vi "REx - Send Command.vi"(0 "Remote Connection Handle in":T2, 7 "Command Data Element in":T1, 11 "error in (no error)":errorcluster) -> (4 "Remote Connection Handle out":T2, 8 "Command Data Element out":T1, 15 "error out":errorcluster)   [LabVIEW 2012, in "REx.lvlib" / "REx - CMD_TEMPLATE.lvclass"]
uses:
  REx - CMD_TEMPLATE.lvclass
  _REx/Components/Remote Connection Session/Typedefs/Session Handle.ctl
  _REx/Components/Remote Connection Session/Remote Connection Session.lvclass
  Data Element/STYP - Command Data Element.ctl
  _REx/Components/REx Command Root/get Command Timed Out.vi
  Data Element/set Command Data Element.vi
  _REx/Components/REx Command Root/set Timeout.vi
  _REx/Components/REx Command Root/set Wait For Response.vi
  Data Element/get Command Data Element.vi
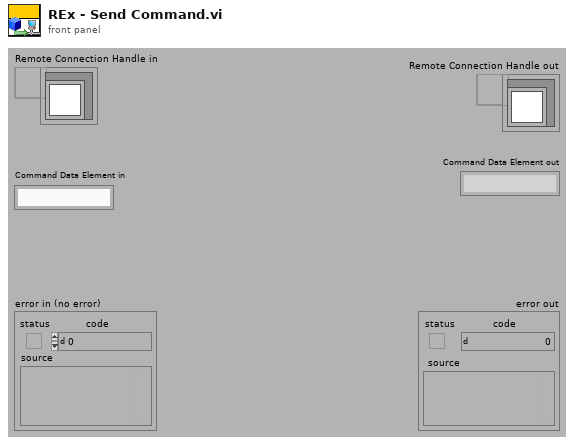
[diagram p1: front panel]
types:
  T1 = typedef "REx.lvlib/REx - CMD_TEMPLATE.lvclass/STYP - Command Data Element.ctl" = string
  T2 = typedef "REx.lvlib/Remote Connection Session.lvclass/Session Handle.ctl" = refnum<data-value>
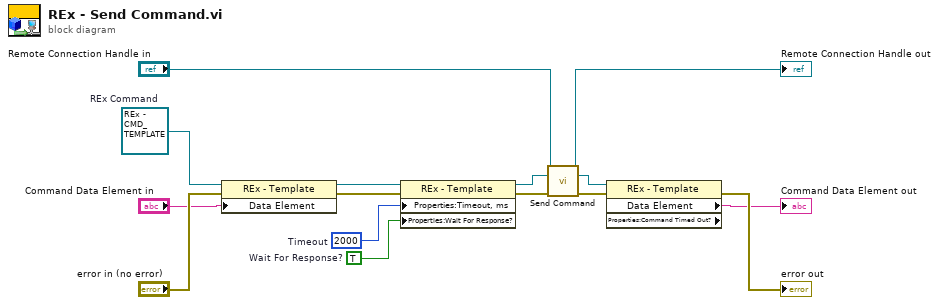
[diagram p0: block diagram]
diagram:
  w1 = TRUE  # Wait For Response?
  w2 = 2000  # Timeout
  w8 = refnum<class "REx - CMD_TEMPLATE.lvclass"> refnum  # REx Command
  n1 = property class="REx - Template"(reference=w8, error in="error in (no error)", "Data Element"="Command Data Element in") -> (reference out=w7:refnum<class "REx - CMD_TEMPLATE.lvclass">, error out=w4:errorcluster)
  n2 = property class="REx - Template"(reference=w7, error in=w4, "Properties:Timeout, ms"=w2, "Properties:Wait For Response?"=w1) -> (reference out=w11:refnum<class "REx - CMD_TEMPLATE.lvclass">, error out=w10:errorcluster)
  n3 = call "Send Command.vi"("Session Handle in"="Remote Connection Handle in", "REx Command in"=w11, "error in (no error)"=w10) -> ("Session Handle out"=→"Remote Connection Handle out":T2, "REx Command out"=w3:refnum<class "REx - CMD_TEMPLATE.lvclass">, "error out"=w9:errorcluster)  [unwired: 10 in]
  n4 = property class="REx - Template" props=["Data Element", "Properties:Command Timed Out?"](reference=w3, error in=w9) -> (error out=→"error out":errorcluster, "Data Element"=→"Command Data Element out":T1)  [unwired: 2 out]
